vi "loadDataToBuffer.vi"(8 "error in (no error)":errorcluster, 11 "DIO64Output in":refnum<class "DIO64Output.lvclass">) -> (0 "error out":errorcluster, 3 "DIO64Output out":refnum<class "DIO64Output.lvclass">)   [LabVIEW 2009, in "Hardware.lvlib" / "Channels.lvlib" / "DIO64Output.lvclass"]
uses:
  DIO64Output.lvclass
  DIO64Output.lvclass/DIO64Output.ctl
panel:
  out "data":u16[][](array[numeric])
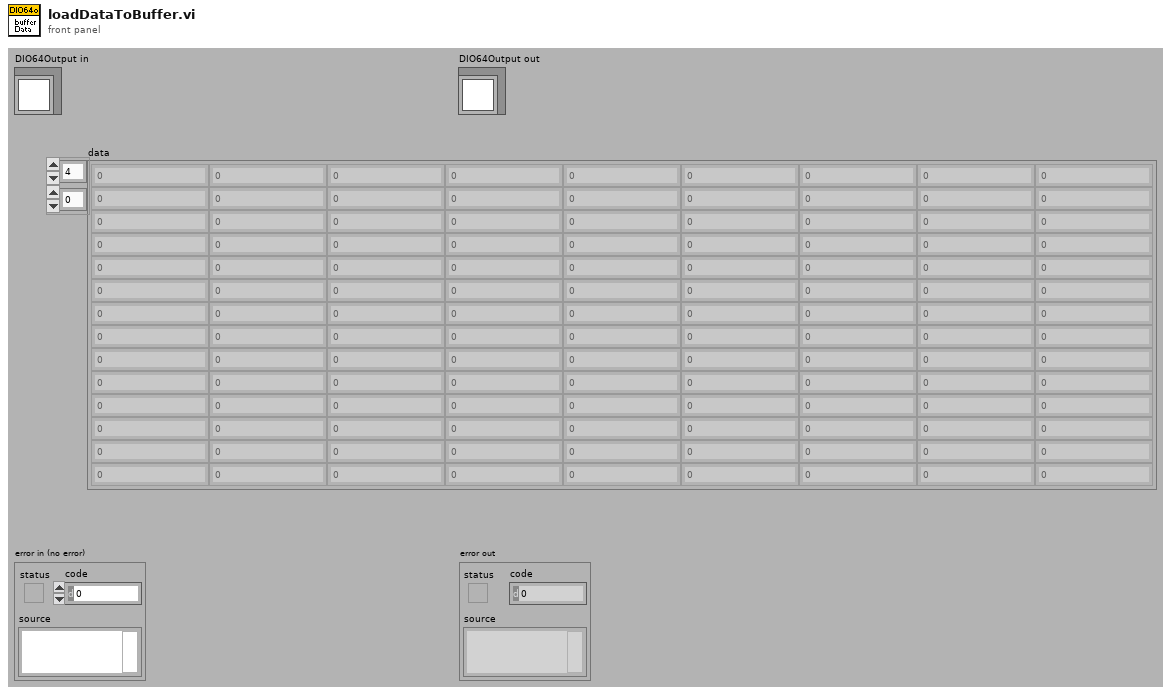
[diagram p1: front panel]
types:
  T1 = cluster{"Timestamps ms":dbl[], "DataPerChannel":dbl[][]}
  T2 = cluster{"Timestamps ms":dbl[], "Bitmap":bool[][]}
  T3 = typedef "DIO64 Out Status.ctl" = cluster{"pktsize":u16, "portCount":u16, "writePtr":u16, "readPtr":u16, "time0":u16, "time1":u16, "fifoSize":u32, "fifo0":u16, "ticks":u32, "flags":u16, "clkControl":u16, "startControl":u16, "stopControl":u16, "AIControl":u32, "AICurrent":u16, "startTime0":u16, "startTime1":u16, "stopTime0":u16, "stopTime1":u16, "cur trans":u32, "cur reps":u32}
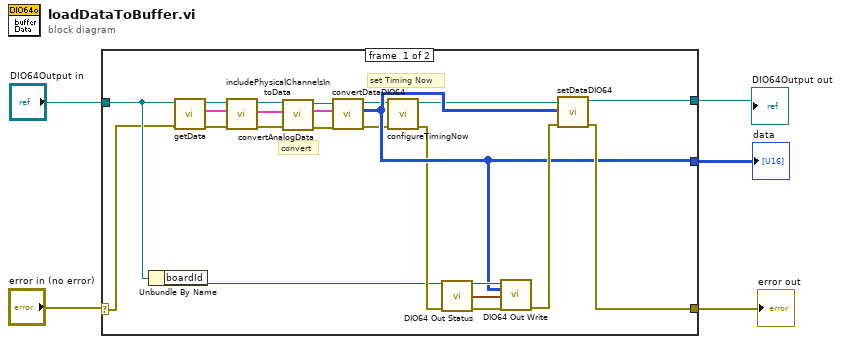
[diagram p0: block diagram]
diagram:
  n1 = case shown="No Error" "error in (no error)" {
    selector: "error in (no error)" -> [w7 w29]
    tunnel: [w25 w30] -> w3
    tunnel: "DIO64Output in" -> [w8 w30]
    tunnel: [w23 w29] -> w2
    tunnel: [w19 _] -> w1
    frame #0 {
      # "set Timing Now"
      # "convert"
      n2 = Unbundle By Name(w8) -> ("boardId"=w6:i32)
      n3 = call-dynamic "getData.vi"("error in (no error)"=w7, "DigitalOutput.lvclass in"=w8) -> ("error out"=w14:errorcluster, "Data"=w10:T1, "DigitalOutput.lvclass out"=w9:refnum<class "DIO64Output.lvclass">)  [unwired: 7 in]
      n4 = call "includePhysicalChannelsIntoData.vi"("error in (no error)"=w14, "Data"=w10, "DIO64Output in"=w9) -> ("error out"=w13:errorcluster, "Data out"=w11:T1, "DIO64Output out"=w12:refnum<class "DIO64Output.lvclass">)  [unwired: 6 in]
      n5 = call "convertAnalogData.vi"("error in (no error)"=w13, "Data"=w11, "DIO64Output in"=w12) -> ("error out"=w20:errorcluster, "digitalData"=w21:T2, "DIO64Output out"=w22:refnum<class "DIO64Output.lvclass">)  [unwired: 6 in]
      n6 = call "convertDataDIO64.vi"("error in (no error)"=w20, "Data"=w21, "DIO64Output in"=w22) -> ("error out"=w17:errorcluster, "data"=w19:u16[][], "DIO64Output out"=w18:refnum<class "DIO64Output.lvclass">)  [unwired: 4 in, 2 out]
      n7 = call "configureTimingNow.vi"("error in (no error)"=w17, "DIO64Output in"=w18) -> ("error out"=w15:errorcluster, "DIO64Output out"=w16:refnum<class "DIO64Output.lvclass">)  [unwired: 8 in]
      n8 = call <userlib>:"DIO64 Out Status.vi"("board in"=w6, "error in (no error)"=w15) -> ("board out"=w28:u16, "Out Status"=w26:T3, "error out"=w27:errorcluster)  [unwired: 10 in, 1 out]
      n9 = call <userlib>:"DIO64 Out Write.vi"("board in"=w28, "data"=w19, "Out Status"=w26, "error in (no error)"=w27) -> ("error out"=w24:errorcluster)  [unwired: 10 in, 1 out]
      n10 = call "setDataDIO64.vi"("error in (no error)"=w24, "data"=w19, "DIO64Output.lvclass in"=w16) -> ("error out"=w23:errorcluster, "DIO64Output.lvclass out"=w25:refnum<class "DIO64Output.lvclass">)  [unwired: 7 in]
    }
    frame #1 {
    }
  }
  "error out" <- w2
  "DIO64Output out" <- w3
  "data" <- w1
